vi "Encode Image (Greyscale).vi"(8 "error in (no error)":errorcluster, 10 "Greyscale Image":T1, 11 "Image to File-Buffer Encoder in":refnum<class "Image to File-Buffer Encoder.lvclass">) -> (0 "error out":errorcluster, 2 "Buffer":string, 3 "Image to File-Buffer Encoder":refnum<class "Image to File-Buffer Encoder.lvclass">)   [LabVIEW 2020, in "image.lvlib" / "Image to File-Buffer Encoder.lvclass"]
uses:
  Image to File-Buffer Encoder.lvclass
  Image to File-Buffer Encoder.lvclass/Image to File-Buffer Encoder.ctl
  c8136873-c742-4257-b221-98e07a73ef51.vi
  Greyscale Image.ctl
  image.lvlib
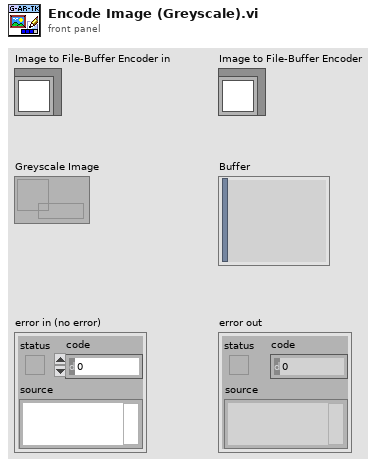
[diagram p1: front panel]
types:
  T1 = typedef "image.lvlib/Greyscale Image.ctl" = refnum<data-value>
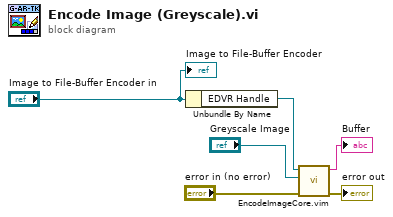
[diagram p0: block diagram]
diagram:
  n1 = Unbundle By Name("Image to File-Buffer Encoder in") -> ("EDVR Handle"=w5:refnum<data-value>)
  n2 = call "EncodeImageCore.vim"("error in (no error)"="error in (no error)", "ARGB Image"="Greyscale Image", "EDVR Handle"=w5) -> ("error out"=→"error out":errorcluster, "Buffer"=→"Buffer":string)  [unwired: 7 in]
  "Image to File-Buffer Encoder" <- "Image to File-Buffer Encoder in"
